vi "Add CellFormat to CellStyleFormats.vi"(8 "error in":errorcluster, 10 "CellFormat in":refnum<k24>, 11 "SpreadsheetDoc in":refnum<k24>) -> (0 "error out":errorcluster, 1 "Index":i32, 2 "CellFormat out":refnum<k24>, 3 "SpreadsheetDoc out":refnum<k24>)   [LabVIEW 2021, in "Open Xml.lvlib"]
uses:
  Open Xml.lvlib
  D:/git/Open-Xml-LabVIEW/dll/DocumentFormat.OpenXml.dll
  dll/DocumentFormat.OpenXml.dll
  D:/git/Open-Xml-LabVIEW/dll/DocumentFormat.OpenXml.Framework.dll
  dll/DocumentFormat.OpenXml.Framework.dll
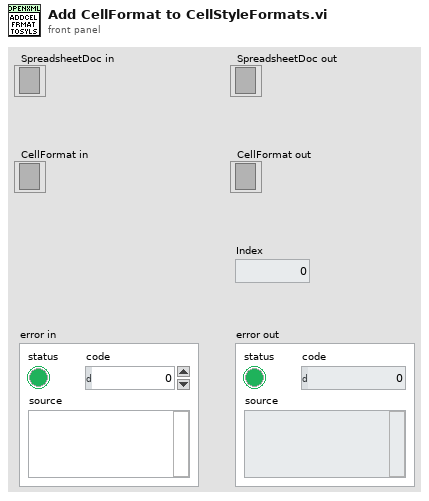
[diagram p1: front panel]
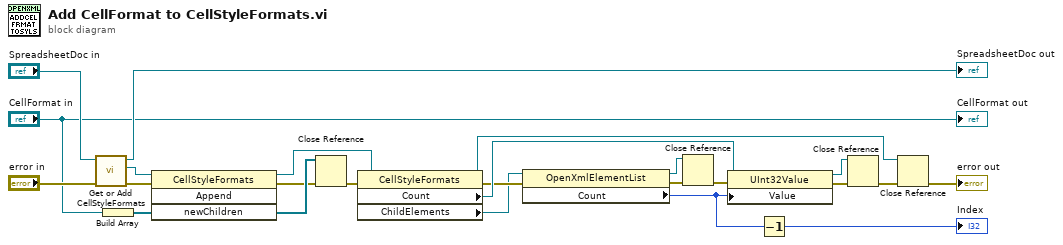
[diagram p0: block diagram]
diagram:
  n1 = call "Get or Add CellStyleFormats.vi"("error in"="error in", "SpreadsheetDoc in"="SpreadsheetDoc in") -> ("error out"=w22:errorcluster, "CellStyleFormats"=w20:refnum<k24>, "SpreadsheetDoc out"=→"SpreadsheetDoc out":refnum<k24>)  [unwired: 7 in]
  n2 = Build Array("CellFormat in") -> (w6:refnum<k24>[])
  n3 = invoke class="CellStyleFormats" method="Append"(reference=w20, error in=w22, "newChildren"=w6) -> (reference out=w17:refnum<k24>, error out=w4:errorcluster, "newChildren"=w5:refnum<k24>[])  [unwired: 1 in, 1 out]
  n4 = Close Reference(reference=w5, error in (no error)=w4) -> (error out=w3:errorcluster)
  n5 = property class="CellStyleFormats"(reference=w17, error in=w3) -> (reference out=w16:refnum<k24>, error out=w11:errorcluster, "Count"=w15:refnum<k24>, "ChildElements"=w10:refnum<k24>)
  n6 = property class="OpenXmlElementList"(reference=w10, error in=w11) -> (reference out=w1:refnum<k24>, error out=w9:errorcluster, "Count"=w8:i32)
  n7 = Close Reference(reference=w1, error in (no error)=w9) -> (error out=w2:errorcluster)
  n8 = property class="UInt32Value"(reference=w15, error in=w2, "Value"=w8) -> (reference out=w12:refnum<k24>, error out=w14:errorcluster)
  n9 = Decrement(x=w8) -> (x-1=→"Index":i32)
  n10 = Close Reference(reference=w12, error in (no error)=w14) -> (error out=w13:errorcluster)
  n11 = Close Reference(reference=w16, error in (no error)=w13) -> (error out=→"error out":errorcluster)
  "CellFormat out" <- "CellFormat in"
